vi "pc.vi"() -> ()   [LabVIEW 2009]
panel:
  out "RAM":i32[](array[numeric])
  out "Symboltable":cluster{"Label":string, "Address":i64}[](array[cluster])
  out "Display":bool[][](array[boolean])
  in  "Stopp":bool
  out "Programm Counter":i64
  out "Programm":string
  out "Stack":i32[](array[numeric])
  in  "Sourcecode":path
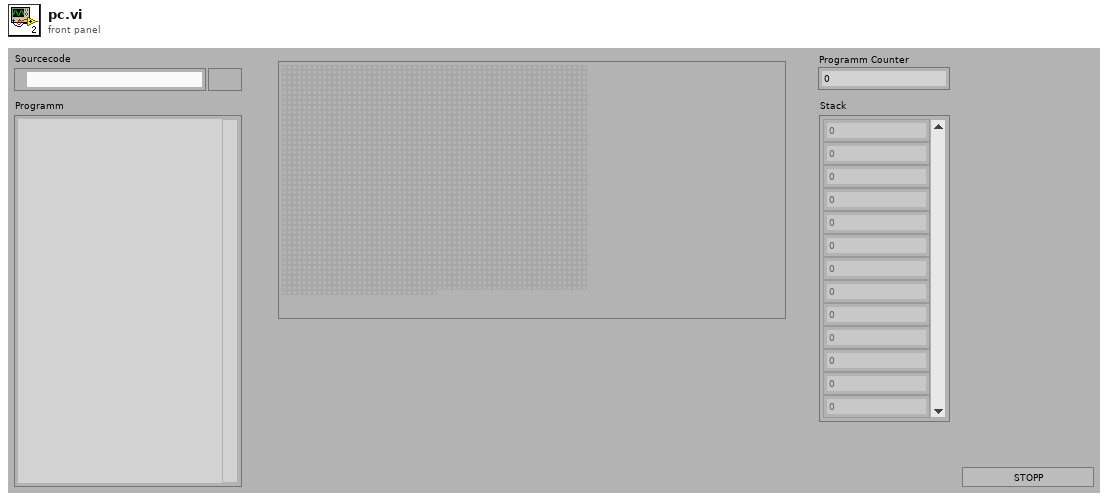
[diagram p1: front panel]
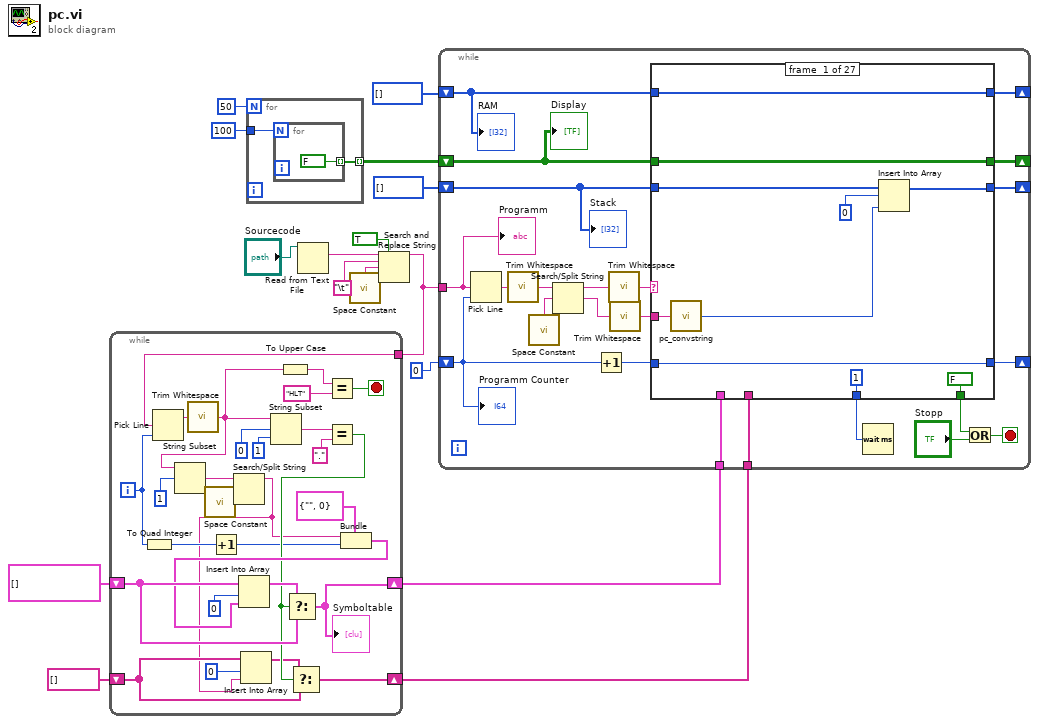
[diagram p0: block diagram]
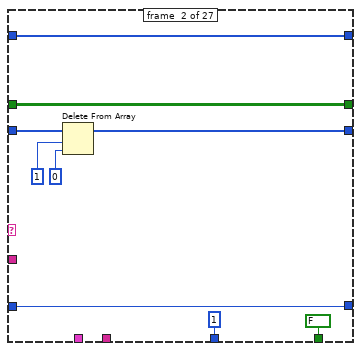
[diagram p2: hidden frame]
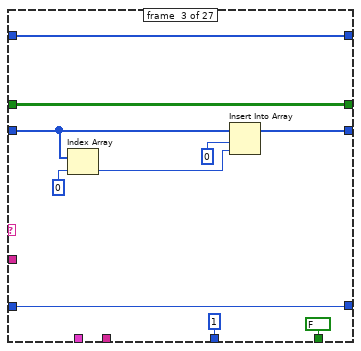
[diagram p3: hidden frame]
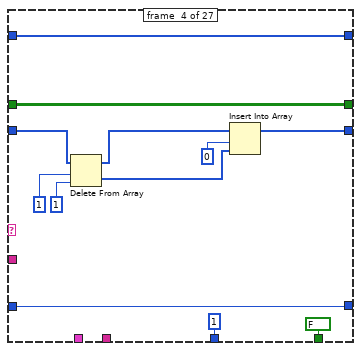
[diagram p4: hidden frame]
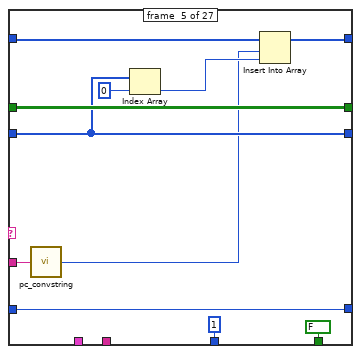
[diagram p5: hidden frame]
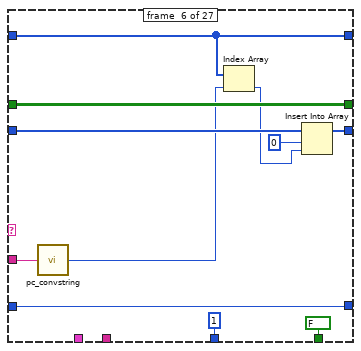
[diagram p6: hidden frame]
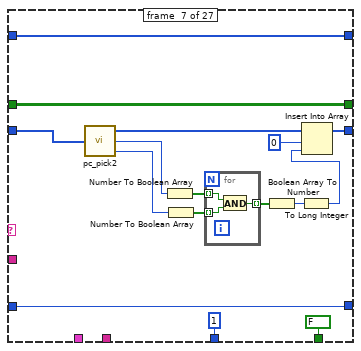
[diagram p7: hidden frame]
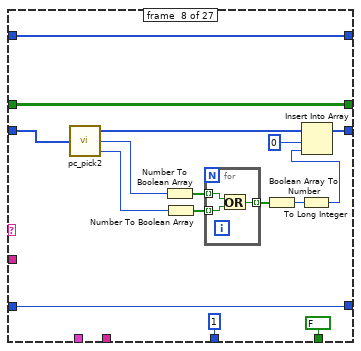
[diagram p8: hidden frame]
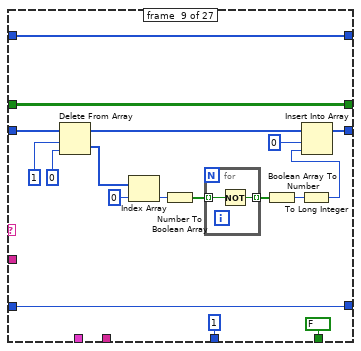
[diagram p9: hidden frame]
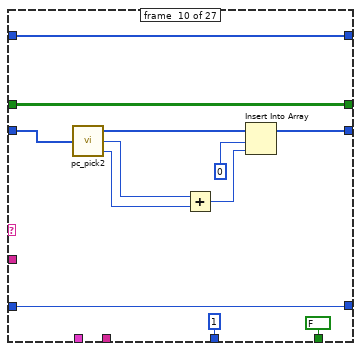
[diagram p10: hidden frame]
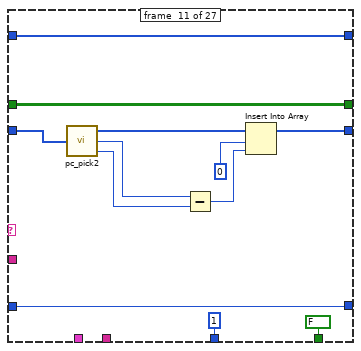
[diagram p11: hidden frame]
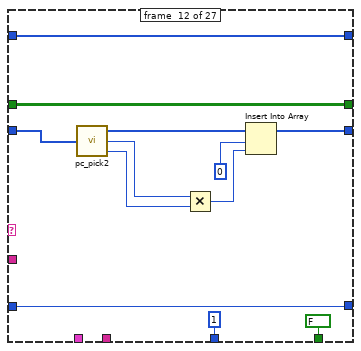
[diagram p12: hidden frame]
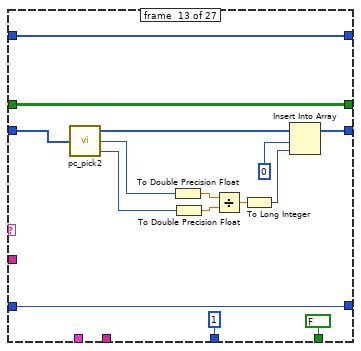
[diagram p13: hidden frame]
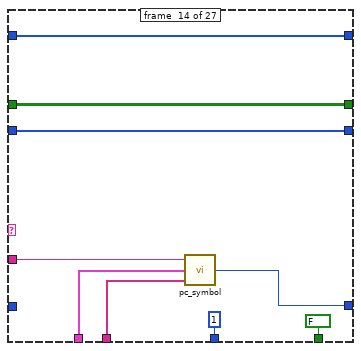
[diagram p14: hidden frame]
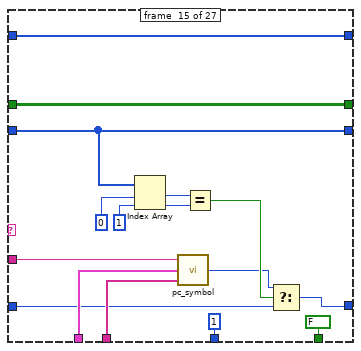
[diagram p15: hidden frame]
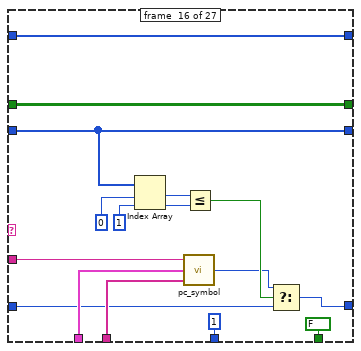
[diagram p16: hidden frame]
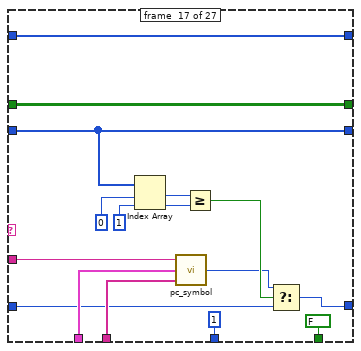
[diagram p17: hidden frame]
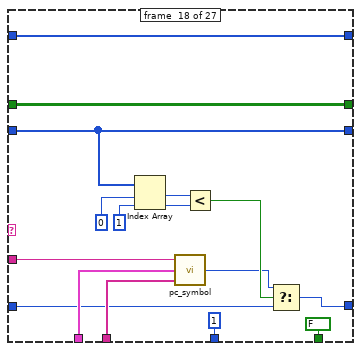
[diagram p18: hidden frame]
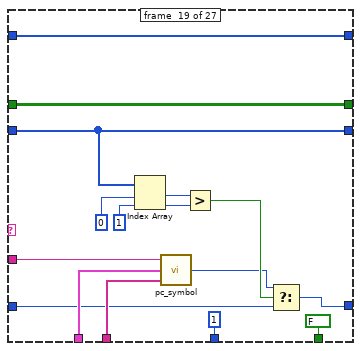
[diagram p19: hidden frame]
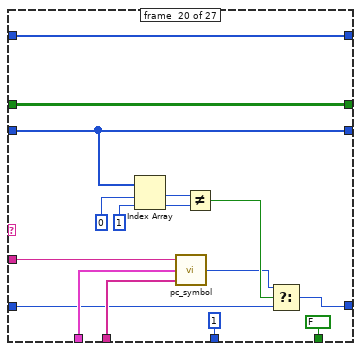
[diagram p20: hidden frame]
diagram:
  n1 = for {
    N: 50 -> [_]
    tunnel: 100 -> [w18]
    tunnel: [w17] -> w12 mode=indexing
    n2 = for {
      N: w18 -> [_]
      tunnel: [FALSE] -> w17 mode=indexing
    }
  }
  n3 = Read from Text File(file (use dialog)="Sourcecode") -> (text=w3:string)  [unwired: 3 in, 3 out]
  n4 = call <vilib>:"Space Constant.vi"() -> ("String"=w4:string)
  n5 = Search and Replace String(replace all?=TRUE ("Alle ersetzen? (F)"), input string=w3, search string="\t", replace string=w4) -> (result string=w2:string)  [unwired: 4 in, 3 out]
  n6 = while {
    tunnel: w2 -> [w47]
    shift-right: [w40] -> w10
    shift-left: cluster{string, i64}[] [] -> [w42]
    shift-right: [w29] -> w8
    shift-left: string[] [] -> [w32]
    i -> [w26]
    stop <- w34 stop-if-true
    n7 = To Quad Integer(1:w26) -> (0:w28:i64)
    n8 = Pick Line(multi-line string=w47, line index=w26) -> (output string=w24:string)  [unwired: 1 in]
    n9 = call <vilib>:"Trim Whitespace.vi"("string"=w24) -> ("trimmed string"=w21:string)  [unwired: 1 in]
    n10 = String Subset(string=w21, offset (0)=1 ("Offset (0)")) -> (substring=w23:string)  [unwired: 1 in]
    n11 = call <vilib>:"Space Constant.vi"() -> ("String"=w25:string)
    n12 = Increment(x=w28) -> (x+1=w27:i64)
    n13 = Search/Split String(string=w23, search string/char (-)=w25) -> (substring before match=w20:string)  [unwired: 1 in, 2 out]
    n14 = Insert Into Array(array=w32, index=0 ("Index"), new element=w20) -> (w31:string[])
    n15 = String Subset(string=w21, offset (0)=0 ("Offset (0)"), length (rest)=1 ("Länge (Rest)")) -> (substring=w37:string)
    n16 = To Upper Case(1:w21) -> (0:w35:string)
    n17 = Equal?(x=w35, y="HLT") -> (x = y?=w34:bool)
    n18 = Equal?(x=w37, y=".") -> (x = y?=w33:bool)
    n19 = Select(t=w31, s=w33, f=w32) -> (s? t:f=w29:string[])
    n20 = Bundle(cluster=cluster{string, i64} {"", 0}, w20, w27) -> (w39:cluster{string, i64})
    n21 = Insert Into Array(array=w42, index=0 ("Index"), new element=w39) -> (w41:cluster{string, i64}[])
    n22 = Select(t=w41, s=w33, f=w42) -> (s? t:f=w40:cluster{string, i64}[])
    "Symboltable" <- w40
  }
  n23 = while {
    shift-right: [w64] -> _
    shift-left: i64 0 -> [w65]
    shift-right: [w66] -> _
    shift-left: i32[] [] -> [w61]
    shift-right: [w60] -> _
    shift-left: w12 -> [w59]
    tunnel: w2 -> [w58]
    tunnel: w10 -> [w57]
    tunnel: w8 -> [w56]
    shift-right: [w53] -> _
    shift-left: i32[] [] -> [w54]
    stop <- w63 stop-if-true
    n24 = Pick Line(multi-line string=w58, line index=w65) -> (output string=w52:string)  [unwired: 1 in]
    n25 = call <vilib>:"Trim Whitespace.vi"("string"=w52) -> ("trimmed string"=w49:string)  [unwired: 1 in]
    n26 = call <vilib>:"Space Constant.vi"() -> ("String"=w69:string)
    n27 = Search/Split String(string=w49, search string/char (-)=w69) -> (substring before match=w68:string, match + rest of string=w67:string)  [unwired: 1 in, 1 out]
    n28 = Increment(x=w65) -> (x+1=w48:i64)
    n29 = call <vilib>:"Trim Whitespace.vi"("string"=w68) -> ("trimmed string"=w51:string)  [unwired: 1 in]
    n30 = call <vilib>:"Trim Whitespace.vi"("string"=w67) -> ("trimmed string"=w50:string)  [unwired: 1 in]
    n31 = case shown="\"BGT\"" w51 {
      tunnel: w50 -> [w74 _ _ _ w114 w125 _ _ _ _ _ _ _ w243 w256 w272 w288 w304 w320 w336 w352 _ w371 _ w402 _ _]
      tunnel: w61 -> [w80 w89 w95 w106 w117 w129 w149 w157 w187 w196 w208 w220 w232 w251 w265 w281 w297 w313 w329 w345 w358 w364 w378 w391 w407 w413 w419]
      tunnel: [w79 w88 w96 w108 w117 w130 w147 w168 w185 w203 w215 w227 w242 w251 w265 w281 w297 w313 w329 w345 w357 w364 w378 w392 w407 w413 w419] -> w66
      tunnel: w48 -> [w71 w81 w90 w100 w112 w123 w134 w153 w172 w192 w204 w216 w228 _ w252 w268 w284 w300 w316 w332 w348 _ w369 w384 w400 w408 w414]
      tunnel: [w71 w81 w90 w100 w112 w123 w134 w153 w172 w192 w204 w216 w228 w246 w267 w283 w299 w315 w331 w347 w349 w361 w369 w384 w400 w408 w414] -> w64
      tunnel: [FALSE FALSE FALSE FALSE FALSE FALSE FALSE FALSE FALSE FALSE FALSE FALSE FALSE FALSE FALSE FALSE FALSE FALSE FALSE FALSE FALSE FALSE FALSE FALSE FALSE TRUE FALSE] -> w62
      tunnel: w59 -> [w75 w84 w98 w110 w121 w132 w138 w160 w175 w199 w211 w223 w235 w249 w262 w278 w294 w310 w326 w342 w359 w367 w381 w396 w405 w411 w417]
      tunnel: [w75 w84 w98 w110 w121 w132 w138 w160 w175 w199 w211 w223 w235 w249 w262 w278 w294 w310 w326 w342 w359 w367 w379 w396 w405 w411 w417] -> w60
      tunnel: w57 -> [_ _ _ _ _ _ _ _ _ _ _ _ _ w248 w255 w271 w287 w303 w319 w335 w351 _ _ _ _ _ _]
      tunnel: w56 -> [_ _ _ _ _ _ _ _ _ _ _ _ _ w247 w254 w270 w286 w302 w318 w334 w350 _ _ _ _ _ _]
      tunnel: [u32 1 u32 1 u32 1 u32 1 u32 1 u32 1 u32 1 u32 1 u32 1 u32 1 u32 1 u32 1 u32 1 u32 1 u32 1 u32 1 u32 1 u32 1 u32 1 u32 1 u32 1 u32 1 u32 1 u32 1 w404 u32 1 u32 1] -> w55
      tunnel: [w72 w82 w91 w101 w118 w128 w135 w158 w173 w197 w209 w221 w233 w244 w257 w273 w289 w305 w321 w337 w353 w365 w372 w385 w403 w409 w415] -> w53
      tunnel: w54 -> [w72 w82 w91 w101 w119 w128 w135 w158 w173 w197 w209 w221 w233 w244 w257 w273 w289 w305 w321 w337 w353 w365 w372 w385 w403 w409 w415]
      frame #0 {
        n32 = call "pc_convstring.vi"("trimmed string"=w74) -> ("number"=w76:i32)
        n33 = Insert Into Array(array=w80, index=0 ("Index"), new element=w76) -> (w79:i32[])
      }
      frame #1 {
        n34 = Delete From Array(array=w89, length=1 ("Länge"), index=0 ("Index")) -> (array with subset deleted=w88:i32[])  [unwired: 1 out]
      }
      frame #2 {
        n35 = Index Array(array=w95, index=0 ("Index")) -> (element=w92:i32)
        n36 = Insert Into Array(array=w95, index=0 ("Index"), new element=w92) -> (w96:i32[])
      }
      frame #3 {
        n37 = Delete From Array(array=w106, length=1 ("Länge"), index=1 ("Index")) -> (deleted portion=w102:i32[], array with subset deleted=w105:i32[])
        n38 = Insert Into Array(array=w105, index=0 ("Index"), new element=w102) -> (w108:i32[])
      }
      frame #4 {
        n39 = call "pc_convstring.vi"("trimmed string"=w114) -> ("number"=w113:i32)
        n40 = Index Array(array=w117, index=0 ("Index")) -> (element=w115:i32)
        n41 = Insert Into Array(array=w119, index=w113, new element=w115) -> (w118:i32[])
      }
      frame #5 {
        n42 = call "pc_convstring.vi"("trimmed string"=w125) -> ("number"=w124:i32)
        n43 = Index Array(array=w128, index=w124) -> (element=w127:i32)
        n44 = Insert Into Array(array=w129, index=0 ("Index"), new element=w127) -> (w130:i32[])
      }
      frame #6 {
        n45 = call "pc_pick2.vi"("original array"=w149) -> ("reduced array"=w148:i32[], "stack element 0"=w145:i32, "stack element 1"=w137:i32)
        n46 = Number To Boolean Array(number=w145) -> (Boolean array=w144:bool[])
        n47 = Number To Boolean Array(number=w137) -> (Boolean array=w143:bool[])
        n48 = for {
          tunnel: w144 -> [w151] mode=indexing
          tunnel: w143 -> [w152] mode=indexing
          tunnel: [w150] -> w142 mode=indexing
          n49 = And(x=w151, y=w152) -> (x .and. y?=w150:bool)
        }
        n50 = Boolean Array To Number(Boolean array=w142) -> (number=w141:u32)
        n51 = To Long Integer(number=w141) -> (32bit integer=w140:i32)
        n52 = Insert Into Array(array=w148, index=0 ("Index"), new element=w140) -> (w147:i32[])
      }
      frame #7 {
        n53 = call "pc_pick2.vi"("original array"=w157) -> ("reduced array"=w156:i32[], "stack element 0"=w155:i32, "stack element 1"=w154:i32)
        n54 = Number To Boolean Array(number=w155) -> (Boolean array=w166:bool[])
        n55 = Number To Boolean Array(number=w154) -> (Boolean array=w165:bool[])
        n56 = for {
          tunnel: w166 -> [w170] mode=indexing
          tunnel: w165 -> [w171] mode=indexing
          tunnel: [w169] -> w164 mode=indexing
          n57 = Or(x=w170, y=w171) -> (x .or. y?=w169:bool)
        }
        n58 = Boolean Array To Number(Boolean array=w164) -> (number=w163:u32)
        n59 = To Long Integer(number=w163) -> (32bit integer=w162:i32)
        n60 = Insert Into Array(array=w156, index=0 ("Index"), new element=w162) -> (w168:i32[])
      }
      frame #8 {
        n61 = Delete From Array(array=w187, length=1 ("Länge"), index=0 ("Index")) -> (deleted portion=w184:i32[], array with subset deleted=w186:i32[])
        n62 = Index Array(array=w184, index=0 ("Index")) -> (element=w181:i32)
        n63 = Number To Boolean Array(number=w181) -> (Boolean array=w180:bool[])
        n64 = for {
          tunnel: w180 -> [w191] mode=indexing
          tunnel: [w190] -> w179 mode=indexing
          n65 = Not(x=w191) -> (.not. x?=w190:bool)
        }
        n66 = Boolean Array To Number(Boolean array=w179) -> (number=w178:u32)
        n67 = To Long Integer(number=w178) -> (32bit integer=w177:i32)
        n68 = Insert Into Array(array=w186, index=0 ("Index"), new element=w177) -> (w185:i32[])
      }
      frame #9 {
        n69 = call "pc_pick2.vi"("original array"=w196) -> ("reduced array"=w195:i32[], "stack element 0"=w194:i32, "stack element 1"=w193:i32)
        n70 = Add(x=w194, y=w193) -> (x+y=w202:i32)
        n71 = Insert Into Array(array=w195, index=0 ("Index"), new element=w202) -> (w203:i32[])
      }
      frame #10 {
        n72 = call "pc_pick2.vi"("original array"=w208) -> ("reduced array"=w207:i32[], "stack element 0"=w206:i32, "stack element 1"=w205:i32)
        n73 = Subtract(x=w206, y=w205) -> (x-y=w214:i32)
        n74 = Insert Into Array(array=w207, index=0 ("Index"), new element=w214) -> (w215:i32[])
      }
      frame #11 {
        n75 = call "pc_pick2.vi"("original array"=w220) -> ("reduced array"=w219:i32[], "stack element 0"=w218:i32, "stack element 1"=w217:i32)
        n76 = Multiply(x=w218, y=w217) -> (x*y=w226:i32)
        n77 = Insert Into Array(array=w219, index=0 ("Index"), new element=w226) -> (w227:i32[])
      }
      frame #12 {
        n78 = call "pc_pick2.vi"("original array"=w232) -> ("reduced array"=w231:i32[], "stack element 0"=w230:i32, "stack element 1"=w229:i32)
        n79 = To Double Precision Float(number=w230) -> (double precision float=w238:dbl)
        n80 = To Double Precision Float(number=w229) -> (double precision float=w237:dbl)
        n81 = Divide(x=w238, y=w237) -> (x/y=w240:dbl)
        n82 = To Long Integer(number=w240) -> (32bit integer=w239:i32)
        n83 = Insert Into Array(array=w231, index=0 ("Index"), new element=w239) -> (w242:i32[])
      }
      frame #13 {
        n84 = call "pc_symbol.vi"("symbols"=w247, "addresses"=w248, "instruction string"=w243) -> ("address"=w246:i64)
      }
      frame #14 {
        n85 = Index Array(array=w265, index #1=0 ("Index"), index #2=1 ("Index")) -> (element #1=w264:i32, element #2=w260:i32)
        n86 = call "pc_symbol.vi"("symbols"=w254, "addresses"=w255, "instruction string"=w256) -> ("address"=w253:i64)
        n87 = Equal?(x=w264, y=w260) -> (x = y?=w266:bool)
        n88 = Select(t=w253, s=w266, f=w252) -> (s? t:f=w267:i64)
      }
      frame #15 {
        n89 = Index Array(array=w281, index #1=0 ("Index"), index #2=1 ("Index")) -> (element #1=w280:i32, element #2=w276:i32)
        n90 = call "pc_symbol.vi"("symbols"=w270, "addresses"=w271, "instruction string"=w272) -> ("address"=w269:i64)
        n91 = Less Or Equal?(x=w280, y=w276) -> (x <= y?=w282:bool)
        n92 = Select(t=w269, s=w282, f=w268) -> (s? t:f=w283:i64)
      }
      frame #16 {
        n93 = Index Array(array=w297, index #1=0 ("Index"), index #2=1 ("Index")) -> (element #1=w296:i32, element #2=w292:i32)
        n94 = call "pc_symbol.vi"("symbols"=w286, "addresses"=w287, "instruction string"=w288) -> ("address"=w285:i64)
        n95 = Greater Or Equal?(x=w296, y=w292) -> (x >= y?=w298:bool)
        n96 = Select(t=w285, s=w298, f=w284) -> (s? t:f=w299:i64)
      }
      frame #17 {
        n97 = Index Array(array=w313, index #1=0 ("Index"), index #2=1 ("Index")) -> (element #1=w312:i32, element #2=w308:i32)
        n98 = call "pc_symbol.vi"("symbols"=w302, "addresses"=w303, "instruction string"=w304) -> ("address"=w301:i64)
        n99 = Less?(x=w312, y=w308) -> (x < y?=w314:bool)
        n100 = Select(t=w301, s=w314, f=w300) -> (s? t:f=w315:i64)
      }
      frame #18 {
        n101 = Index Array(array=w329, index #1=0 ("Index"), index #2=1 ("Index")) -> (element #1=w328:i32, element #2=w324:i32)
        n102 = call "pc_symbol.vi"("symbols"=w318, "addresses"=w319, "instruction string"=w320) -> ("address"=w317:i64)
        n103 = Greater?(x=w328, y=w324) -> (0:w330:bool)
        n104 = Select(t=w317, s=w330, f=w316) -> (s? t:f=w331:i64)
      }
      frame #19 {
        n105 = Index Array(array=w345, index #1=0 ("Index"), index #2=1 ("Index")) -> (element #1=w344:i32, element #2=w340:i32)
        n106 = call "pc_symbol.vi"("symbols"=w334, "addresses"=w335, "instruction string"=w336) -> ("address"=w333:i64)
        n107 = Not Equal?(x=w344, y=w340) -> (x != y?=w346:bool)
        n108 = Select(t=w333, s=w346, f=w332) -> (s? t:f=w347:i64)
      }
      frame #20 {
        n109 = call "pc_symbol.vi"("symbols"=w350, "addresses"=w351, "instruction string"=w352) -> ("address"=w349:i64)
        n110 = To Long Integer(number=w348) -> (32bit integer=w356:i32)
        n111 = Insert Into Array(array=w358, index=0 ("Index"), new element=w356) -> (w357:i32[])
      }
      frame #21 {
        n112 = Index Array(array=w364, index=0 ("Index")) -> (element=w362:i32)
        n113 = To Quad Integer(1:w362) -> (0:w361:i64)
      }
      frame #22 {
        n114 = call "pc_convstring.vi"("trimmed string"=w371) -> ("number"=w370:i32)
        n115 = Equal?(x=w370, y=1) -> (x = y?=w376:bool)
        n116 = Index Array(array=w378, index #1=1 ("Index"), index #2=0 ("Index")) -> (element #1=w380:i32, element #2=w374:i32)
        n117 = Replace Array Subset(array=w381, new element=w376, index (row)=w380, index (col)=w374) -> (w379:bool[][])
      }
      frame #23 {
        n118 = Index Array(array=w391, index #1=1 ("Index"), index #2=0 ("Index")) -> (element #1=w395:i32, element #2=w394:i32)
        n119 = Index Array(array=w396, index (row)=w395, index (col)=w394) -> (element=w390:bool)
        n120 = Select(t=1, s=w390, f=0) -> (s? t:f=w389:i32)
        n121 = Insert Into Array(array=w391, index=0 ("Index"), new element=w389) -> (w392:i32[])
      }
      frame #24 {
        n122 = call "pc_convstring.vi"("trimmed string"=w402) -> ("number"=w401:i32)
        n123 = To Unsigned Long Integer(number=w401) -> (unsigned 32bit integer=w404:u32)
      }
      frame #25 {
      }
      frame #26 {
      }
    }
    n124 = Wait (ms)(milliseconds to wait=w55) -> ()  [unwired: 1 out]
    n125 = Or(x=w62, y="Stopp") -> (x .or. y?=w63:bool)
    "Programm Counter" <- w65
    "Programm" <- w58
    "Stack" <- w61
    "Display" <- w59
    "RAM" <- w54
  }
